vi "EOL Create AI Channel Task.vi"() -> (0 "Error Out":errorcluster, 3 "Analog Input Task":refnum<k21>)   [LabVIEW 2018]
uses:
  02.Type Def's/Scalling Configuration Control.ctl
  02.Type Def's/AIO Channel Configuration Control.ctl
  <vilib>/DAQmx/create/scale.llb/DAQmx Create Scale (Linear).vi
  <vilib>/DAQmx/create/channels.llb/DAQmx Create Channel (AI-Voltage-Basic).vi
  <vilib>/DAQmx/create/channels.llb/DAQmx Create Channel (AI-Temperature-Thermocouple).vi
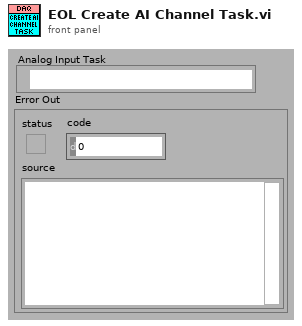
[diagram p1: front panel]
types:
  T1 = typedef "Scalling Configuration Control.ctl" = cluster{"name":string, "slope":dbl}
  T2 = typedef "AIO Channel Configuration Control.ctl" = cluster{"input terminal configuration":i32, "minimum value":dbl, "maximum value":dbl, "physical channel":string, "channel name":string, "units":i32, "custom scale name":string, "type":enum16{"voltage", "thermocouple", "Amps"}}
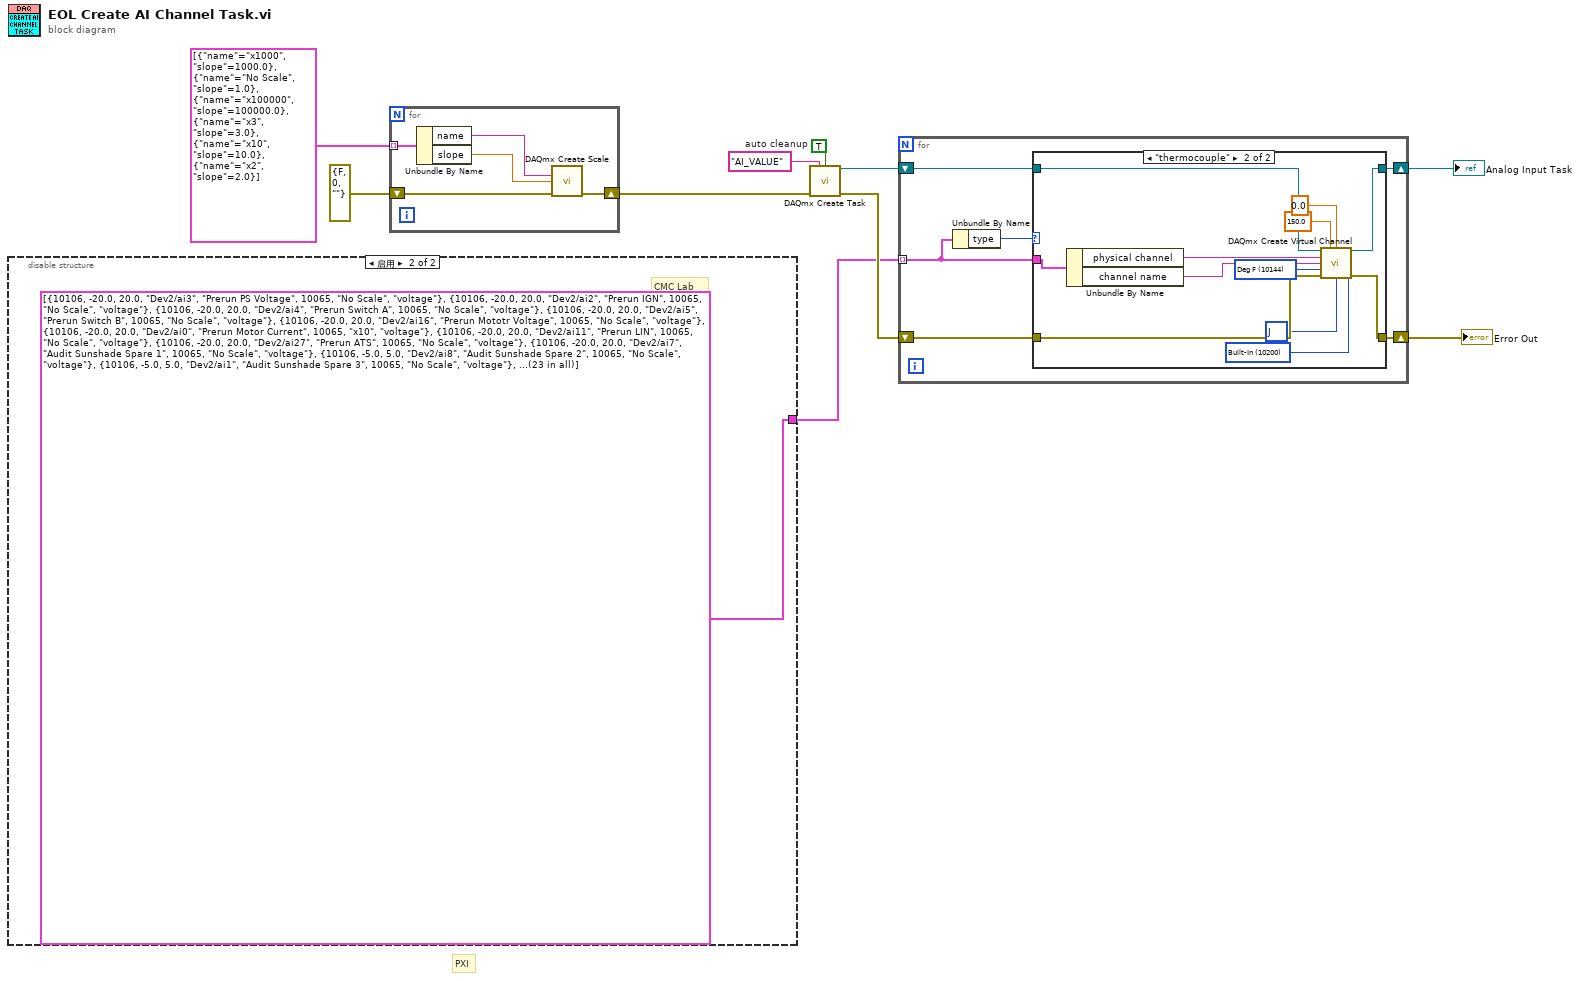
[diagram p0: block diagram]
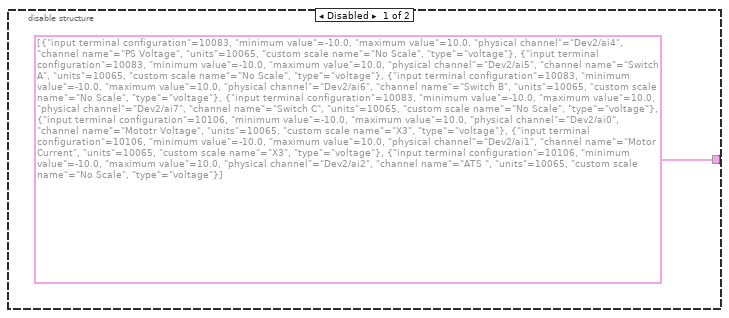
[diagram p2: hidden frame]
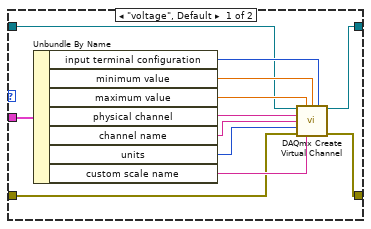
[diagram p3: hidden frame]
diagram:
  w10 = TRUE  # auto cleanup
  # "PXI"
  n1 = disable-structure shown="启用" {
    disable-tunnel: [T2[] [{"input terminal configuration"=10083, "minimum value"=-10.0, "maximum value"=10.0, "physical channel"="Dev2/ai4", "channel name"="PS Voltage", "units"=10065, "custom scale name"="No Scale", "type"=enum."voltage"}, {"input terminal configuration"=10083, "minimum value"=-10.0, "maximum value"=10.0, "physical channel"="Dev2/ai5", "channel name"="Switch A", "units"=10065, "custom scale name"="No Scale", "type"=enum."voltage"}, {"input terminal configuration"=10083, "minimum value"=-10.0, "maximum value"=10.0, "physical channel"="Dev2/ai6", "channel name"="Switch B", "units"=10065, "custom scale name"="No Scale", "type"=enum."voltage"}, {"input terminal configuration"=10083, "minimum value"=-10.0, "maximum value"=10.0, "physical channel"="Dev2/ai7", "channel name"="Switch C", "units"=10065, "custom scale name"="No Scale", "type"=enum."voltage"}, {"input terminal configuration"=10106, "minimum value"=-10.0, "maximum value"=10.0, "physical channel"="Dev2/ai0", "channel name"="Mototr Voltage", "units"=10065, "custom scale name"="X3", "type"=enum."voltage"}, {"input terminal configuration"=10106, "minimum value"=-10.0, "maximum value"=10.0, "physical channel"="Dev2/ai1", "channel name"="Motor Current", "units"=10065, "custom scale name"="X3", "type"=enum."voltage"}, {"input terminal configuration"=10106, "minimum value"=-10.0, "maximum value"=10.0, "physical channel"="Dev2/ai2", "channel name"="ATS ", "units"=10065, "custom scale name"="No Scale", "type"=enum."voltage"}] T2[] [{"input terminal configuration"=10106, "minimum value"=-20.0, "maximum value"=20.0, "physical channel"="Dev2/ai3", "channel name"="Prerun PS Voltage", "units"=10065, "custom scale name"="No Scale", "type"=enum."voltage"}, {"input terminal configuration"=10106, "minimum value"=-20.0, "maximum value"=20.0, "physical channel"="Dev2/ai2", "channel name"="Prerun IGN", "units"=10065, "custom scale name"="No Scale", "type"=enum."voltage"}, {"input terminal configuration"=10106, "minimum value"=-20.0, "maximum value"=20.0, "physical channel"="Dev2/ai4", "channel name"="Prerun Switch A", "units"=10065, "custom scale name"="No Scale", "type"=enum."voltage"}, {"input terminal configuration"=10106, "minimum value"=-20.0, "maximum value"=20.0, "physical channel"="Dev2/ai5", "channel name"="Prerun Switch B", "units"=10065, "custom scale name"="No Scale", "type"=enum."voltage"}, {"input terminal configuration"=10106, "minimum value"=-20.0, "maximum value"=20.0, "physical channel"="Dev2/ai16", "channel name"="Prerun Mototr Voltage", "units"=10065, "custom scale name"="No Scale", "type"=enum."voltage"}, {"input terminal configuration"=10106, "minimum value"=-20.0, "maximum value"=20.0, "physical channel"="Dev2/ai0", "channel name"="Prerun Motor Current", "units"=10065, "custom scale name"="x10", "type"=enum."voltage"}, {"input terminal configuration"=10106, "minimum value"=-20.0, "maximum value"=20.0, "physical channel"="Dev2/ai11", "channel name"="Prerun LIN", "units"=10065, "custom scale name"="No Scale", "type"=enum."voltage"}, {"input terminal configuration"=10106, "minimum value"=-20.0, "maximum value"=20.0, "physical channel"="Dev2/ai27", "channel name"="Prerun ATS", "units"=10065, "custom scale name"="No Scale", "type"=enum."voltage"}, {"input terminal configuration"=10106, "minimum value"=-20.0, "maximum value"=20.0, "physical channel"="Dev2/ai7", "channel name"="Audit Sunshade Spare 1", "units"=10065, "custom scale name"="No Scale", "type"=enum."voltage"}, {"input terminal configuration"=10106, "minimum value"=-5.0, "maximum value"=5.0, "physical channel"="Dev2/ai8", "channel name"="Audit Sunshade Spare 2", "units"=10065, "custom scale name"="No Scale", "type"=enum."voltage"}, {"input terminal configuration"=10106, "minimum value"=-5.0, "maximum value"=5.0, "physical channel"="Dev2/ai1", "channel name"="Audit Sunshade Spare 3", "units"=10065, "custom scale name"="No Scale", "type"=enum."voltage"}, {"input terminal configuration"=10106, "minimum value"=-5.0, "maximum value"=5.0, "physical channel"="Dev2/ai6", "channel name"="Audit Sunshade Spare 4", "units"=10065, "custom scale name"="No Scale", "type"=enum."voltage"}, {"input terminal configuration"=10106, "minimum value"=-20.0, "maximum value"=20.0, "physical channel"="Dev2/ai9", "channel name"="Audit PS Voltage", "units"=10065, "custom scale name"="No Scale", "type"=enum."voltage"}, {"input terminal configuration"=10106, "minimum value"=-20.0, "maximum value"=20.0, "physical channel"="Dev2/ai10", "channel name"="Audit Sunshade Current", "units"=10065, "custom scale name"="x10", "type"=enum."voltage"}, {"input terminal configuration"=10106, "minimum value"=-5.0, "maximum value"=5.0, "physical channel"="Dev2/ai15", "channel name"="Sunshade Hall A", "units"=10065, "custom scale name"="No Scale", "type"=enum."voltage"}, {"input terminal configuration"=10106, "minimum value"=-10.0, "maximum value"=10.0, "physical channel"="Dev2/ai17", "channel name"="Sunshade Hall B", "units"=10065, "custom scale name"="No Scale", "type"=enum."voltage"}, {"input terminal configuration"=10106, "minimum value"=-20.0, "maximum value"=20.0, "physical channel"="Dev2/ai12", "channel name"="Repair PS Voltage", "units"=10065, "custom scale name"="No Scale", "type"=enum."voltage"}, {"input terminal configuration"=10106, "minimum value"=-20.0, "maximum value"=20.0, "physical channel"="Dev2/ai13", "channel name"="Repair IGN", "units"=10065, "custom scale name"="No Scale", "type"=enum."voltage"}, {"input terminal configuration"=10106, "minimum value"=-20.0, "maximum value"=20.0, "physical channel"="Dev2/ai14", "channel name"="Repair Switch A", "units"=10065, "custom scale name"="No Scale", "type"=enum."voltage"}, {"input terminal configuration"=10106, "minimum value"=-20.0, "maximum value"=20.0, "physical channel"="Dev2/ai18", "channel name"="Repair Switch B", "units"=10065, "custom scale name"="No Scale", "type"=enum."voltage"}, {"input terminal configuration"=10106, "minimum value"=-20.0, "maximum value"=20.0, "physical channel"="Dev2/ai19", "channel name"="Repair Motor Voltage", "units"=10065, "custom scale name"="No Scale", "type"=enum."voltage"}, {"input terminal configuration"=10106, "minimum value"=-20.0, "maximum value"=20.0, "physical channel"="Dev2/ai20", "channel name"="Repair Motor Current", "units"=10065, "custom scale name"="No Scale", "type"=enum."voltage"}, {"input terminal configuration"=10106, "minimum value"=-20.0, "maximum value"=20.0, "physical channel"="Dev2/ai21", "channel name"="Repair LIN", "units"=10065, "custom scale name"="No Scale", "type"=enum."voltage"}]] -> w2
    frame Disabled {
    }
    frame Enabled {
      # "CMC Lab"
    }
  }
  n2 = for {
    shift-right: [w17] -> w9
    shift-left: errorcluster {"status"=FALSE, "code"=0, "source"=""} ("error out") -> [w16]
    tunnel: T1[] [{"name"="x1000", "slope"=1000.0}, {"name"="No Scale", "slope"=1.0}, {"name"="x100000", "slope"=100000.0}, {"name"="x3", "slope"=3.0}, {"name"="x10", "slope"=10.0}, {"name"="x2", "slope"=2.0}] -> [w15] mode=indexing
    n3 = Unbundle By Name(w15) -> ("name"=w14:string, "slope"=w13:dbl)
    n4 = call-poly <vilib>:"DAQmx Create Scale.vi"("name"=w14, "slope"=w13, "error in"=w16) -> ("error out"=w17:errorcluster)  [unwired: 3 in, 9 out]
  }
  n5 = call <vilib>:"DAQmx Create Task.vi"("new task name"="AI_VALUE", "auto cleanup"=w10, "error in"=w9) -> ("task out"=w8:refnum<k21>, "error out"=w7:errorcluster)  [unwired: 2 in, 9 out]
  n6 = for {
    tunnel: w2 -> [w19] mode=indexing
    shift-right: [w22] -> w4
    shift-left: w8 -> [w23]
    shift-right: [w20] -> w3
    shift-left: w7 -> [w21]
    n7 = Unbundle By Name(w19) -> ("type"=w18:enum16{"voltage", "thermocouple", "Amps"})
    n8 = case shown="\"thermocouple\"" w18 {
      tunnel: w19 -> [w35 w47]
      tunnel: w23 -> [w27 w44]
      tunnel: [w26 w43] -> w22
      tunnel: w21 -> [w25 w42]
      tunnel: [w24 w41] -> w20
      frame "voltage", Default {
        n9 = Unbundle By Name(w35) -> ("input terminal configuration"=w34:i32, "minimum value"=w33:dbl, "maximum value"=w32:dbl, "physical channel"=w31:string, "channel name"=w30:string, "units"=w29:i32, "custom scale name"=w28:string)
        n10 = call-poly <vilib>:"DAQmx Create Virtual Channel.vi"("task in"=w27, "maximum value"=w32, "minimum value"=w33, "input terminal configuration"=w34, "physical channels"=w31, "name to assign"=w30, "units"=w29, "error in"=w25, "custom scale name"=w28) -> ("task out"=w26:refnum<k21>, "error out"=w24:errorcluster)  [unwired: 5 out]
      }
      frame "thermocouple" {
        w36 = 10144 items=["Deg C"=10143, "Deg F"=10144, "Kelvins"=10325, "Deg R"=10145, "From Custom Scale"=10065] ("units")
        w39 = 10200 items=["Built-In"=10200, "Constant Value"=10116, "Channel"=10113] ("cjc source")
        w40 = 10072 items=["J"=10072, "K"=10073, "N"=10077, "R"=10082, "S"=10085, "T"=10086, "B"=10047, "E"=10055] ("thermocouple type")
        n11 = Unbundle By Name(w47) -> ("physical channel"=w46:string, "channel name"=w45:string)
        n12 = call-poly <vilib>:"DAQmx Create Virtual Channel.vi"("task in"=w44, "maximum value"=150.0, "minimum value"=0.0, "physical channels"=w46, "cjc source"=w39, "name to assign"=w45, "units"=w36, "error in"=w42, "thermocouple type"=w40) -> ("task out"=w43:refnum<k21>, "error out"=w41:errorcluster)  [unwired: 4 in, 1 out]
      }
    }
  }
  "Analog Input Task" <- w4
  "Error Out" <- w3
